vi "Set up FOV control.vi"(8 "error in (no error)":errorcluster) -> (0 "error out":errorcluster)   [LabVIEW 2017]
uses:
  <vilib>/Utility/miscctls.llb/LVStringsAndValuesArrayTypeDef_SGL.ctl
  Global Variables/gl_UI Ctrl Refs.vi
  FOV code/Typedefs/FOV FGV states.ctl
panel:
  in  "Field of View":sgl(ring)=4.35 items=["175 um"=4.35, "250 um"=5.7, "350 um"=8.7]
  out "Strings And Values []":T1=[{"String"="175 µm", "Value"=4.35}, {"String"="235 µm", "Value"=5.6}, {"String"="350 µm", "Value"=8.7}]
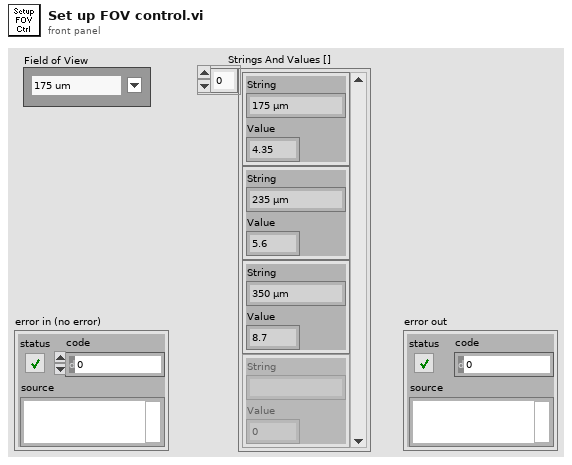
[diagram p1: front panel]
types:
  T1 = typedef "LVStringsAndValuesArrayTypeDef_SGL.ctl" = cluster{"String":string, "Value":sgl}[]
  T2 = typedef "UI ctrl refs cluster.ctl" = cluster{"Top level VI path":path, "Top level VI ref":refnum<vi>, "User menu ref":refnum<k9>, "Sub Panel control":refnum<vi>, "Imaging Param Tab":refnum<vi>, "Occurrence-Start drivers":refnum<k4>, "Occurrence-Speed logging initialised":refnum<k4>, "Occurrence-XYZ stage initialised":refnum<k4>, "Exit button":refnum<vi>, "Status ind":refnum<vi>, "Set as origin":refnum<vi>, "Speed Logging":refnum<vi>, "Time Lapse":refnum<vi>, "Live Imaging":refnum<vi>, "AOL Z Stack":refnum<vi>, "Motor Z Stack":refnum<vi>, "Funct Acq button":refnum<vi>, "Hard Shutter":refnum<vi>, "Virtual Shutter":refnum<vi>, "Laser Power":refnum<vi>, "AOL Mode":refnum<vi>, "Frame Size":refnum<vi>, "Field of View":refnum<vi>, "Dwell Time":refnum<vi>, "Zoom":refnum<vi>, "AOL Z":refnum<vi>, "Objective":refnum<vi>, "Axis":refnum<vi>, "Paths & Names":refnum<vi>, "Experiment folder path (ind.)":refnum<vi>, "Last State (Ind.)":refnum<vi>, "Averages":refnum<vi>, "Angle (degrees)":refnum<vi>, "X centre":refnum<vi>, "Y centre":refnum<vi>, "Plane Mode":refnum<vi>, "# Planes":refnum<vi>, "Z Start":refnum<vi>, "Z Stop":refnum<vi>, "Z Step":refnum<vi>, "PMT 1":refnum<vi>, "PMT 2":refnum<vi>, "Stage XYZ Position":refnum<vi>, "Pockels@Z Start":refnum<vi>, "Pockels@Z Stop":refnum<vi>, "Obtain Z Start":refnum<vi>, "Obtain Z Stop":refnum<vi>, "Live stim.trig.period":refnum<vi>, "Live stim.trig.enable":refnum<vi>, "Movement Correction":refnum<vi>, "Load Reference Image":refnum<vi>, "XY Stage Move":refnum<vi>, "MovCor Cluster":refnum<vi>, "RefDAQParam":refnum<vi>, "Funct. Acq. Pockels Modulation":refnum<vi>, "Background MovCor":refnum<vi>, "Ref Laser Power":refnum<vi>, "Enable Video Recording":refnum<vi>, "Video Record-Live Imaging":refnum<vi>, "Video Record-Funct acq":refnum<vi>, "Reference Source":refnum<vi>, "AOL Z-stack Chirps Ready (ind)":refnum<vi>, "Target time between mov.cor. ref triggers (ms)":refnum<vi>, "Funct. Acq. Ref frame save":refnum<vi>, "Tracking button":refnum<vi>, "Show ref plots window":refnum<vi>, "Center freq ind (nm)":refnum<vi>, "Pickup mode (ind)":refnum<vi>, "Logging queue (ind)":refnum<vi>, "Back aperture power (ind.)":refnum<vi>, "Power after objective (ind.)":refnum<vi>, "Switch user":refnum<vi>, "Ls1 Conn. Status":refnum<vi>, "Ls1Tuning Status":refnum<vi>, "Ls1 Faults":refnum<vi>, "Ls1 Connection":refnum<vi>, "Ls1 Mode":refnum<vi>, "Ls1 POWER [mW]":refnum<vi>, "Ls1Shutter":refnum<vi>, "Ls1 Wavelength":refnum<vi>, "Ls1 Note":refnum<vi>, "Ls1 Confirm Wav":refnum<vi>, "Ls1 PreChrp Prism1":refnum<vi>, "Ls1 PreChrp Prism2":refnum<vi>, "Ls1 wav top Ind":refnum<vi>, "Ls1 power top Ind":refnum<vi>, "Ls1 Pump peak Hold":refnum<vi>, "Ls1 Status Ind":refnum<vi>, "Ls1 wav cancel":refnum<vi>, "Experiment Type":refnum<vi>, "Biology Information":refnum<vi>}
  T3 = typedef "FOV FGV states.ctl" = enum16{"Load from file", "Read FGV", "Update section name", "Delete section", "Add section", "Cleanup ini file"}
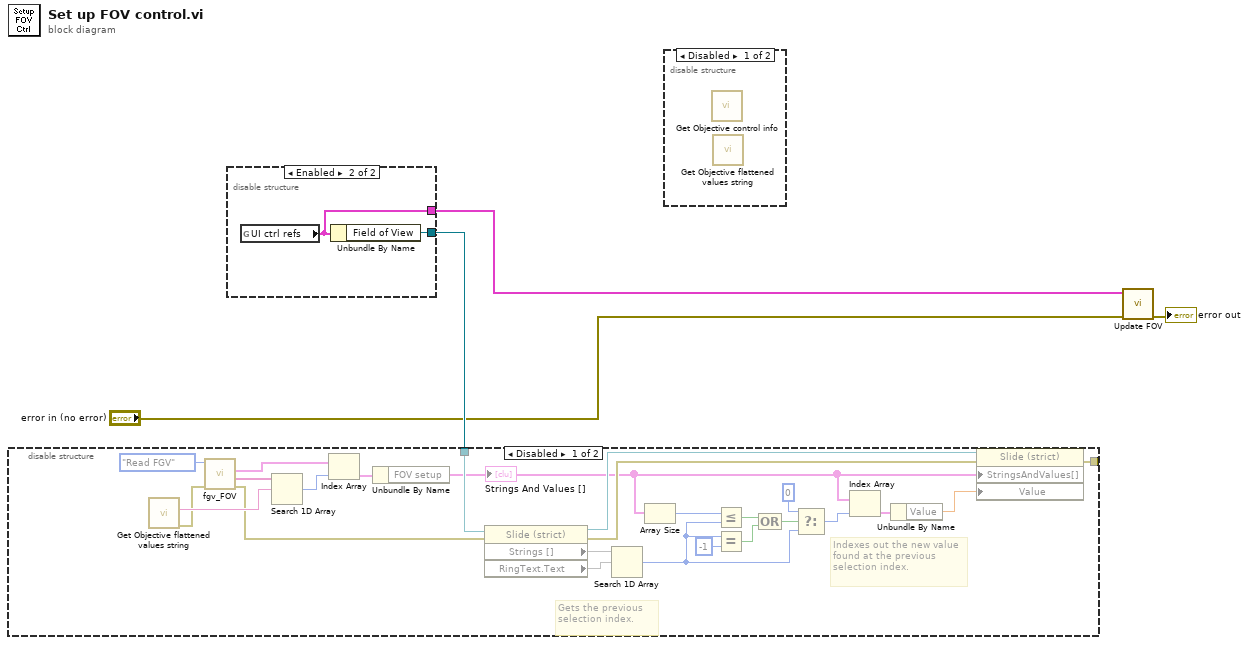
[diagram p0: block diagram]
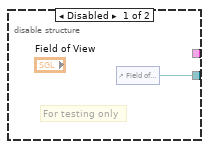
[diagram p4: hidden frame]
diagram:
  n1 = disable-structure shown="Enabled" {
    disable-tunnel: [w5 w7] -> w2
    disable-tunnel: [_ w6] -> w3
    frame Disabled {
      # "For testing only"
      n2 = control-ref of="Field of View"() -> (w5:refnum<vi>)
    }
    frame Enabled {
      n3 = global read "gl_UI Ctrl Refs.vi" "UI ctrl refs"() -> (w6:T2)
      n4 = Unbundle By Name(w6) -> ("Field of View"=w7:refnum<vi>)
    }
  }
  n5 = disable-structure shown="Disabled" {
    disable-tunnel: w2 -> [w23 _]
    disable-tunnel: [w8 _] -> _
    frame Disabled {
      # "Indexes out the new value found at the previous selection index."
      # "Gets the previous selection index."
      n6 = call "Get Objective flattened values string.vi"() -> ("error out"=w10:errorcluster, "Objective.Value"=w11:string)  [unwired: 9 in, 1 out]
      n7 = call "fgv_FOV.vi"("error in"=w10, "Function"=FOV_FGV_states."Read FGV") -> ("error out"=w9:errorcluster, "Objectives (section names)"=w16:string[], "Data (Format B)"=w14:cluster{"FOV setup":T1}[])  [unwired: 6 in, 1 out]
      n8 = Search 1D Array(1D array=w16, element=w11) -> (index of element=w15:i32)  [unwired: 1 in]
      n9 = Index Array(array=w14, index=w15) -> (element=w13:cluster{"FOV setup":T1})
      n10 = Unbundle By Name(w13) -> ("FOV setup"=w12:T1)
      "Strings And Values []" <- w12
      n11 = property on="Property Node" class="Slide (strict)"(reference=w23, error in=w9) -> (reference out=w29:refnum<vi>, error out=w28:errorcluster, "Strings []"=w32, "RingText.Text"=w31)
      n12 = Search 1D Array(1D array=w32, element=w31) -> (index of element=w22:i32)  [unwired: 1 in]
      n13 = Array Size(array=w12) -> (size(s)=w26:i32)
      n14 = Less Or Equal?(x=w26, y=w22) -> (x <= y?=w20:bool)
      n15 = Equal?(x=w22, y=-1) -> (x = y?=w18:bool)
      n16 = Compound Arithmetic op=OR(w20, w18) -> (w19:bool)
      n17 = Select(t=0, s=w19, f=w22) -> (s? t:f=w25:i32)
      n18 = Index Array(array=w12, index=w25) -> (element=w30:cluster{"String":string, "Value":sgl})
      n19 = Unbundle By Name(w30) -> ("Value"=w27:sgl)
      n20 = property on="Property Node" class="Slide (strict)"(reference=w29, error in=w28, "StringsAndValues[]"=w12, "Value"=w27) -> (error out=w8:errorcluster)  [unwired: 1 out]
    }
    frame Enabled {
    }
  }
  n21 = disable-structure shown="Disabled" {
    frame Disabled {
      n22 = call "Get Objective control info.vi"() -> ()  [unwired: 7 in, 5 out]
      n23 = call "Get Objective flattened values string.vi"() -> ()  [unwired: 9 in, 3 out]
    }
    frame Enabled {
    }
  }
  n24 = call "Update FOV.vi"("error in (no error)"="error in (no error)", "UI ctrl refs"=w3) -> ("error out"=→"error out":errorcluster)  [unwired: 9 in]
